vi "Map Actual Values.vi"(0 "Actual Values Array In":dbl[](array[numeric])) -> (6 "Actual Values":map{string, dbl}(c390), 8 "Pump Actuals":T2 {"Status Byte" max=65; "Actual Air Temperature [°C]" min=0.0 max=64.255; "Actual Electronic Temperature [°C]" min=0.0 max=64.255; "Actual Voltage [V]" min=0.0 max=64.255; "Actual Current [A]" min=0.0 max=64.255; "Actual Mass Flow [kg/h]" min=0.0 max=64.255}, 10 "Status Word":T1)   [LabVIEW 2025, in "phlair-busch-can-bus.lvlib"]
uses:
  phlair-busch-can-bus.lvlib
  PumpActuals.ctl
  PumpStatus.ctl
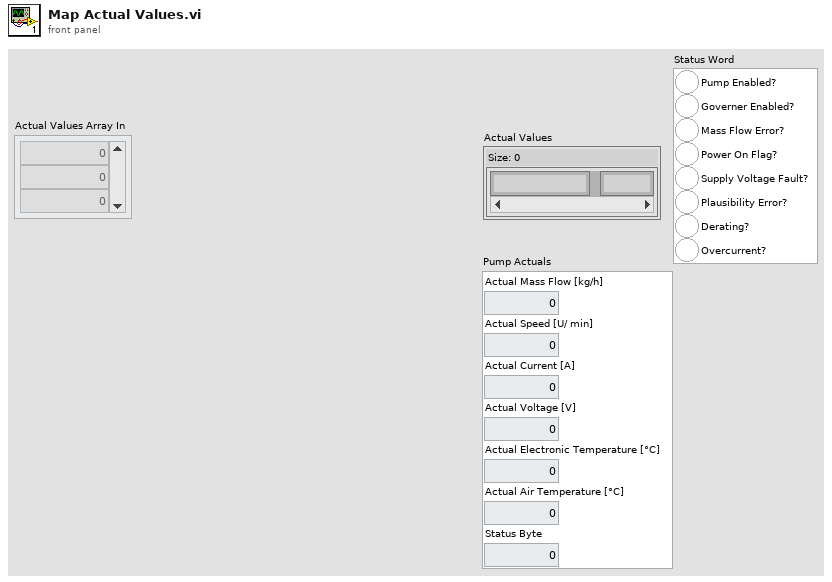
[diagram p1: front panel]
types:
  T1 = typedef "phlair-busch-can-bus.lvlib/PumpStatus.ctl" = cluster{"Pump Enabled?":bool, "Governer Enabled?":bool, "Mass Flow Error?":bool, "Power On Flag?":bool, "Supply Voltage Fault?":bool, "Plausibility Error?":bool, "Derating?":bool, "Overcurrent?":bool}
  T2 = typedef "phlair-busch-can-bus.lvlib/PumpActuals.ctl" = cluster{"Actual Mass Flow [kg/h]":dbl, "Actual Speed [U/ min]":dbl, "Actual Current [A]":dbl, "Actual Voltage [V]":dbl, "Actual Electronic Temperature [°C]":dbl, "Actual Air Temperature [°C]":dbl, "Status Byte":u8}
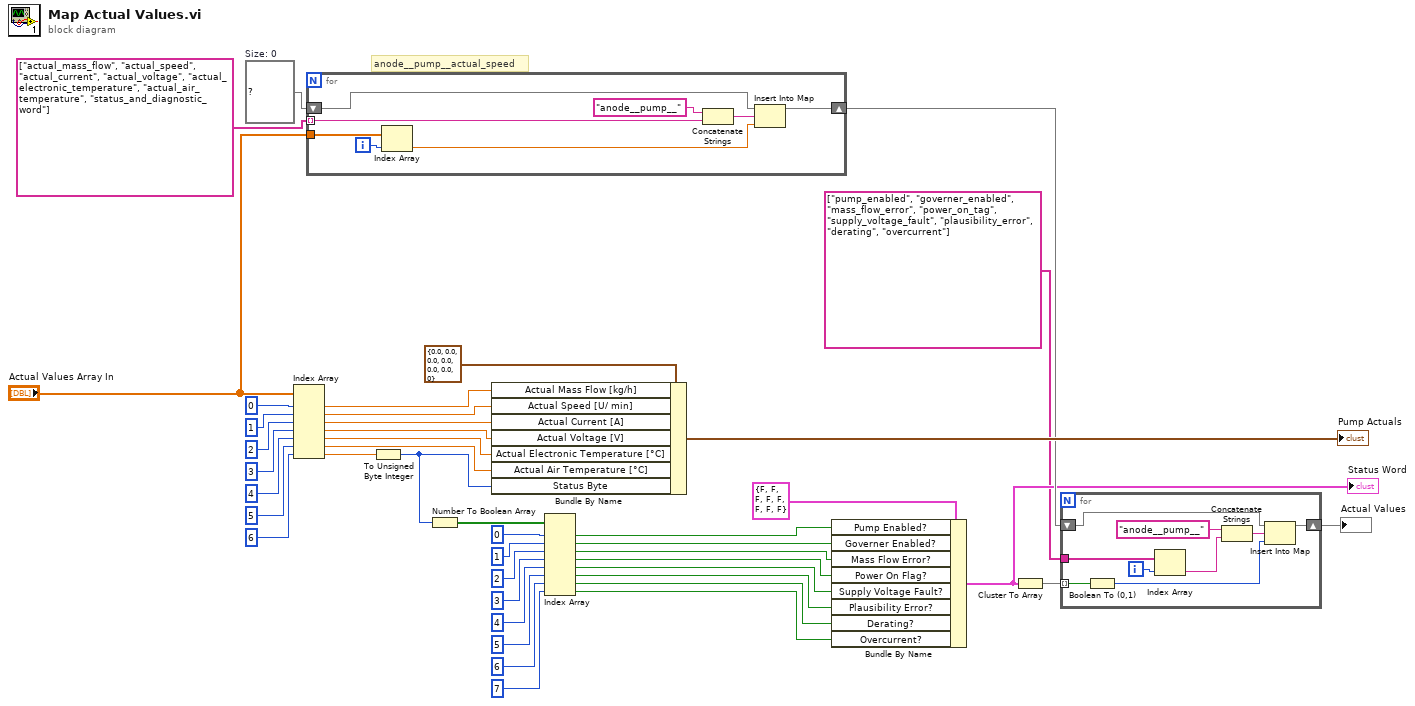
[diagram p0: block diagram]
diagram:
  w42 = map{string, dbl} {}  # Size: 0
  # "anode__pump__actual_speed"
  n1 = Index Array(array="Actual Values Array In", index #1=0 ("index"), index #2=1 ("index"), index #3=2 ("index"), index #4=3 ("index"), index #5=4 ("index"), index #6=5 ("index"), index #7=6 ("index")) -> (element #1=w36:dbl, element #2=w35:dbl, element #3=w33:dbl, element #4=w31:dbl, element #5=w29:dbl, element #6=w27:dbl, element #7=w25:dbl)
  n2 = for {
    tunnel: string[] ["actual_mass_flow", "actual_speed", "actual_current", "actual_voltage", "actual_electronic_temperature", "actual_air_temperature", "status_and_diagnostic_word"] -> [w45] mode=indexing
    tunnel: "Actual Values Array In" -> [w51]
    shift-right: [w48] -> w5
    shift-left: w42 -> [w47]
    i -> [w50]
    n3 = Index Array(array=w51, index=w50) -> (element=w49:dbl)
    n4 = Concatenate Strings("anode__pump__", w45) -> (w44:string)
    n5 = Insert Into Map(map in=w47, key=w44, value=w49) -> (map out=w48:map{string, dbl})  [unwired: 2 out]
  }
  n6 = To Unsigned Byte Integer(number=w25) -> (unsigned 8bit integer=w24:u8)
  n7 = Number To Boolean Array(number=w24) -> (Boolean array=w23:bool[])
  n8 = Bundle By Name(cluster=T2 {"Actual Mass Flow [kg/h]"=0.0, "Actual Speed [U/ min]"=0.0, "Actual Current [A]"=0.0, "Actual Voltage [V]"=0.0, "Actual Electronic Temperature [°C]"=0.0, "Actual Air Temperature [°C]"=0.0, "Status Byte"=0} ("Pump Actuals"), "Actual Mass Flow [kg/h]"=w36, "Actual Speed [U/ min]"=w35, "Actual Current [A]"=w33, "Actual Voltage [V]"=w31, "Actual Electronic Temperature [°C]"=w29, "Actual Air Temperature [°C]"=w27, "Status Byte"=w24) -> (→"Pump Actuals":T2)
  n9 = Index Array(array=w23, index #1=0 ("index"), index #2=1 ("index"), index #3=2 ("index"), index #4=3 ("index"), index #5=4 ("index"), index #6=5 ("index"), index #7=6 ("index"), index #8=7 ("index")) -> (element #1=w21:bool, element #2=w12:bool, element #3=w11:bool, element #4=w10:bool, element #5=w9:bool, element #6=w8:bool, element #7=w7:bool, element #8=w6:bool)
  n10 = Bundle By Name(cluster=T1 {"Pump Enabled?"=FALSE, "Governer Enabled?"=FALSE, "Mass Flow Error?"=FALSE, "Power On Flag?"=FALSE, "Supply Voltage Fault?"=FALSE, "Plausibility Error?"=FALSE, "Derating?"=FALSE, "Overcurrent?"=FALSE} ("Pump Status"), "Pump Enabled?"=w21, "Governer Enabled?"=w12, "Mass Flow Error?"=w11, "Power On Flag?"=w10, "Supply Voltage Fault?"=w9, "Plausibility Error?"=w8, "Derating?"=w7, "Overcurrent?"=w6) -> (w3:T1)
  "Status Word" <- w3
  n11 = Cluster To Array(cluster=w3) -> (array=w2:bool[])
  n12 = for {
    shift-right: [w59] -> w4
    shift-left: w5 -> [w58]
    tunnel: w2 -> [w56] mode=indexing
    tunnel: string[] ["pump_enabled", "governer_enabled", "mass_flow_error", "power_on_tag", "supply_voltage_fault", "plausibility_error", "derating", "overcurrent"] -> [w57]
    i -> [w60]
    n13 = Boolean To (0,1)(Boolean=w56) -> (0, 1=w55:i16)
    n14 = Index Array(array=w57, index=w60) -> (element=w53:string)
    n15 = Concatenate Strings("anode__pump__", w53) -> (w52:string)
    n16 = Insert Into Map(map in=w58, key=w52, value=w55) -> (map out=w59:map{string, dbl})  [unwired: 2 out]
  }
  "Actual Values" <- w4
